vi "IV_config_DMM.vi"(8 "error in (no error)":errorcluster, 11 "Input parameters":T1={"Measurement type"=enum."Debug", "Sensor type"=enum."HPK_8in_271ch", "Identifier"="test.txt", "Open after execution?"=FALSE, "Plot after execution?"=FALSE, "Display channel"=0, "Voltage Delay (s)"=0.5, "Switch Delay (s)"=0.01, "VISA resource name source"="", "VISA resource name DMM"="", "VISA resource name LCR"="", "Compliance  Level (A)"=10.0, "Voltage Limit (V)"=1000.0, "Data storage location"="", "Scan voltages"="", "Use source as DMM?"=FALSE, "LCR signal frequenzy (Hz)"=10.0, "DMM device"=enum."Keithley2001", "Sampling number"=1, "Use env. sensors on"=enum."Sensirion sht1x/7x", "Switchboard Handle"=0, "Use Switchboard"=FALSE, "LCR signal voltage (V)"=10000.0, "Repeat"=1, "Scan voltages IV"="", "Scan voltages CV"="", "Hex pad numbers?"=FALSE, "Set measurement type"=enum."Debug", "Custom pad scan"="", "IV voltage Delay (s)"=0.5, "CV voltage Delay (s)"=0.5, "Needle measurement?"=FALSE, "Comments"="test.txt", "LCR signal frequenzy (kHz)"=10.0, "Compliance  Level (uA)"=10.0, "Open Correction Array"=array2304x3[6912 elements], "Current set voltage"=0.0, "Last set voltage"=0.0, "Current channel"=0, "Last OpenCorrection index"=-1, "Total curr/vltg every x steps"=10, "Current channel iteration"=0, "No CV corrections"=FALSE, "Mapfile"="", "Corrfile"="", "IV voltage file"=path "", "CV voltage file"=path "", "IV Switch Delay (s)"=0.01, "CV Switch Delay (s)"=0.01, "Invert polarity"=FALSE, "Set debug dirs"=FALSE, "Is n on p"=FALSE, "Source interlock?"=TRUE, "Voltage file used?"=FALSE, "Pad mask"="", "Mask pad above (uA)"=1.0, "LCR device"=enum."LCR_E4980", "Source device"=enum."Source_2410"} {"CV Switch Delay (s)" format="%#_13g"; "IV Switch Delay (s)" format="%#_13g"; "Last set voltage" format="%#_13g"; "Current set voltage" format="%#_13g"; "CV voltage Delay (s)" format="%#_13g"; "IV voltage Delay (s)" format="%#_13g"; "Voltage Limit (V)" format="%#_13g"; "Voltage Delay (s)" format="%#_13g"; "Switch Delay (s)" format="%#_13g"}) -> (0 "error out":errorcluster)   [LabVIEW 2016]
doc: "Sets configuration for DMM."
uses:
  input_params.ctl
  <instrlib>/ke2001/KE2001.LLB/Keith 2001 Reset / Preset.vi
  <instrlib>/Keithley 2450/Keithley 2450.lvlib
  <instrlib>/Keithley 6517/Keithley 6517.lvlib
  <instrlib>/Keithley 648X Series/Keithley 648X Series.lvlib
panel:
  out "VISA resource name out":refnum<visa-resource-name>
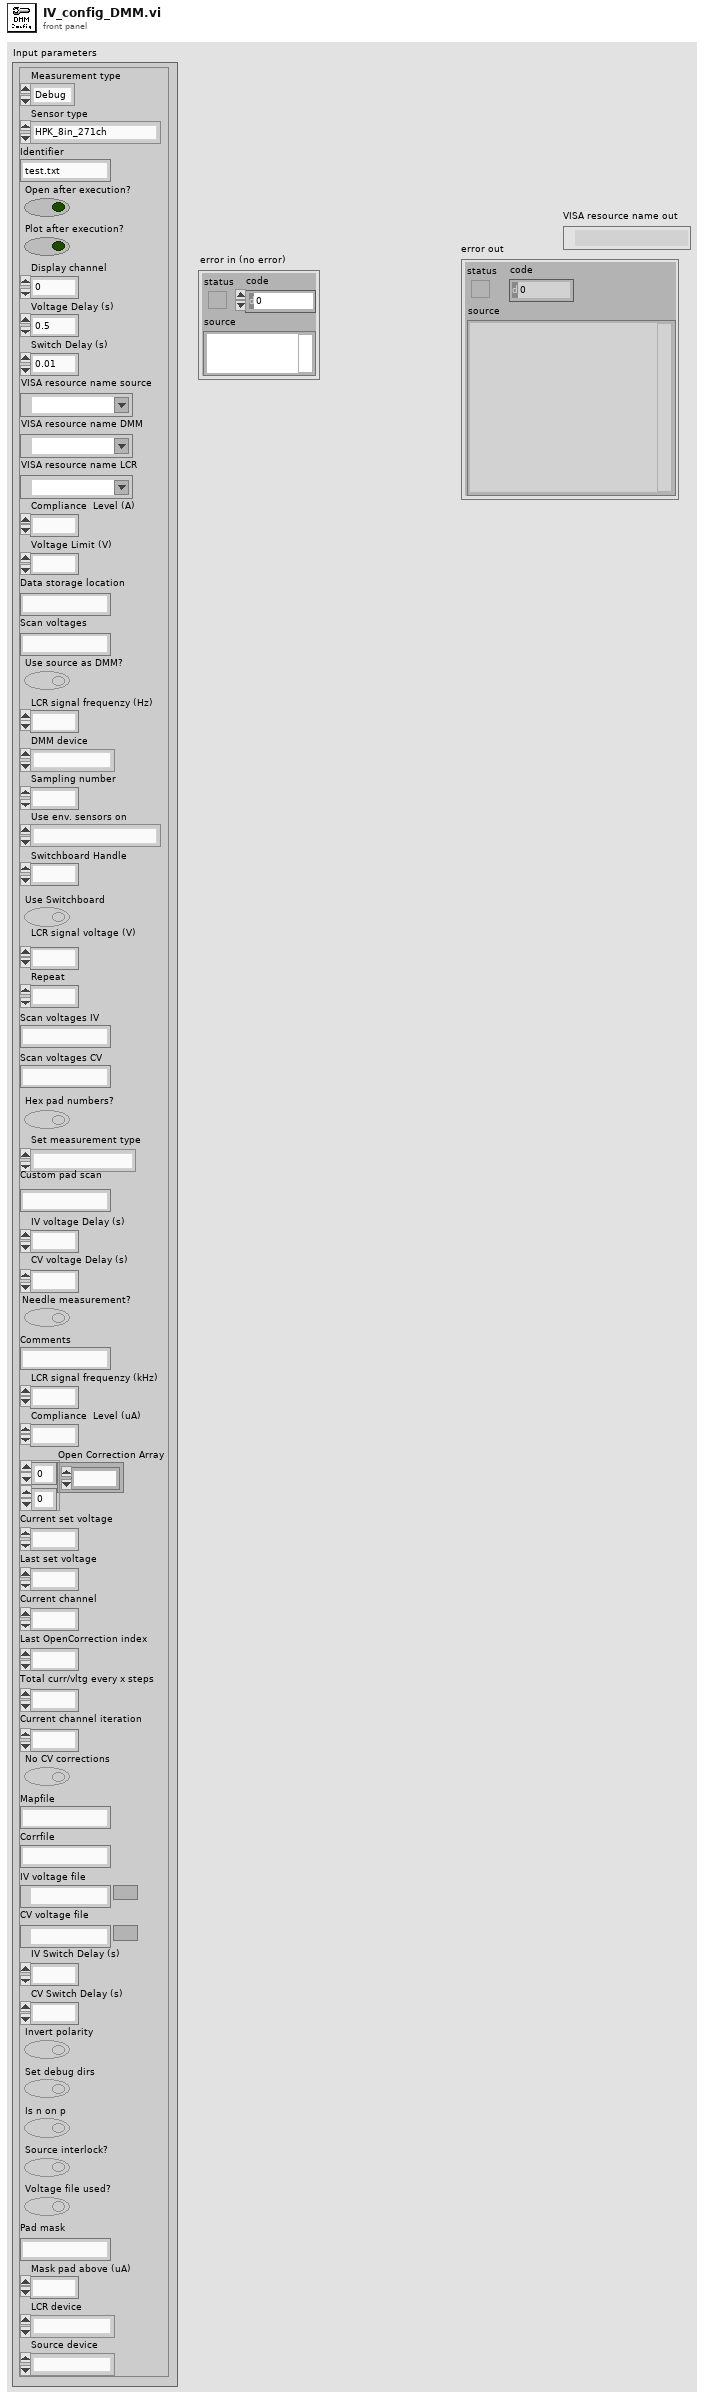
[diagram p1: front panel]
types:
  T1 = typedef "input_params.ctl" = cluster{"Measurement type":enum16{"IV", "CV", "Debug", "Test_contact"}, "Sensor type":enum16{"HPK_6in_135ch", "HPK_8in_271ch", "IFX_8in_256ch", "Diode", "HPK_6in_239ch", "Full_Matrix", "HPK_8in_271ch_full", "HPK_8in_198ch", "LumiCal"}, "Identifier":string, "Open after execution?":bool, "Plot after execution?":bool, "Display channel":i32, "Voltage Delay (s)":dbl, "Switch Delay (s)":dbl, "VISA resource name source":refnum<visa-resource-name>, "VISA resource name DMM":refnum<visa-resource-name>, "VISA resource name LCR":refnum<visa-resource-name>, "Compliance  Level (A)":dbl, "Voltage Limit (V)":dbl, "Data storage location":string, "Scan voltages":string, "Use source as DMM?":bool, "LCR signal frequenzy (Hz)":dbl, "DMM device":enum16{"Keithley2001", "Keithley2450", "Keithley2410", "Keithley6485", "Keithley6487", "Keithley6517"}, "Sampling number":i32, "Use env. sensors on":enum16{"Sensirion sht1x/7x", "Switch Matrix", "Probecard"}, "Switchboard Handle":u32, "Use Switchboard":bool, "LCR signal voltage (V)":dbl, "Repeat":i32, "Scan voltages IV":string, "Scan voltages CV":string, "Hex pad numbers?":bool, "Set measurement type":enum16{"IV", "CV", "Debug", "Test_contact", "IV+CV"}, "Custom pad scan":string, "IV voltage Delay (s)":dbl, "CV voltage Delay (s)":dbl, "Needle measurement?":bool, "Comments":string, "LCR signal frequenzy (kHz)":dbl, "Compliance  Level (uA)":dbl, "Open Correction Array":dbl[][], "Current set voltage":dbl, "Last set voltage":dbl, "Current channel":i32, "Last OpenCorrection index":i32, "Total curr/vltg every x steps":i32, "Current channel iteration":i32, "No CV corrections":bool, "Mapfile":string, "Corrfile":string, "IV voltage file":path, "CV voltage file":path, "IV Switch Delay (s)":dbl, "CV Switch Delay (s)":dbl, "Invert polarity":bool, "Set debug dirs":bool, "Is n on p":bool, "Source interlock?":bool, "Voltage file used?":bool, "Pad mask":string, "Mask pad above (uA)":dbl, "LCR device":enum16{"LCR_E4980", "AGILENT_4263X"}, "Source device":enum16{"Source_2410", "Source_6487"}}
  T2 = enum16{"Keithley2001", "Keithley2450", "Keithley2410", "Keithley6485", "Keithley6487", "Keithley6517"}
  T3 = enum16{"Auto On", "2e-9", "2e-8", "2e-7", "2e-6", "2e-5", "2e-4", "2e-3", "2e-2"}
  T4 = cluster{"error":bool, "code":i32, "source":string}
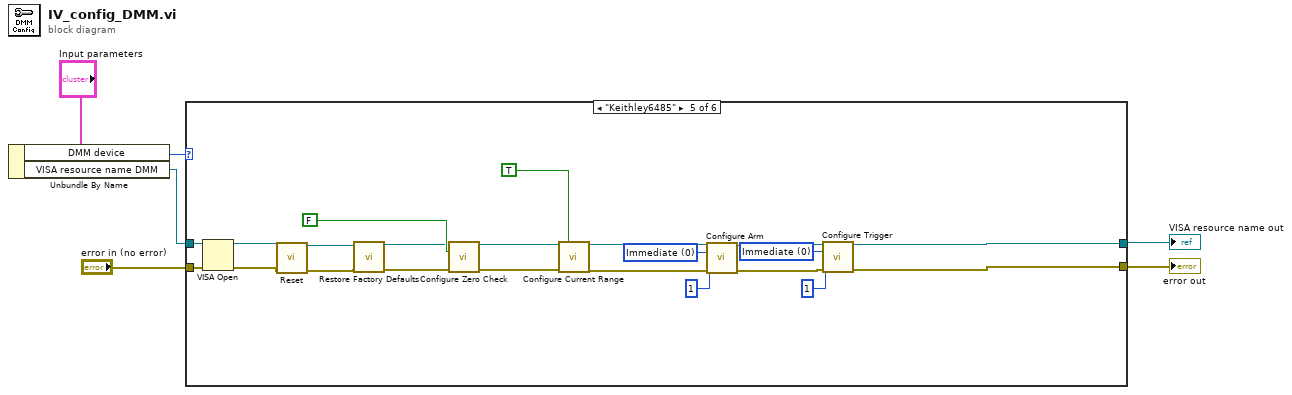
[diagram p0: block diagram]
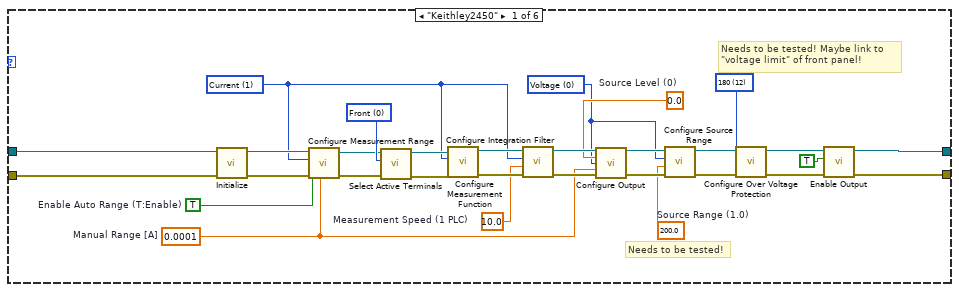
[diagram p2: hidden frame]
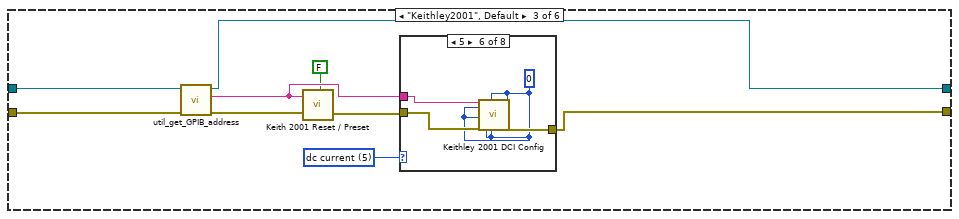
[diagram p4: hidden frame]
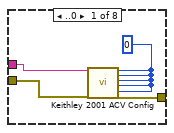
[diagram p5: hidden frame]
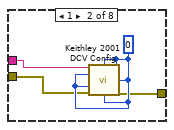
[diagram p6: hidden frame]
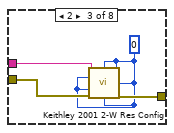
[diagram p7: hidden frame]
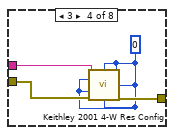
[diagram p8: hidden frame]
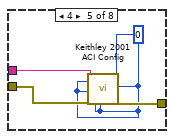
[diagram p9: hidden frame]
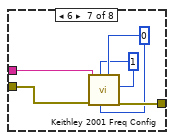
[diagram p10: hidden frame]
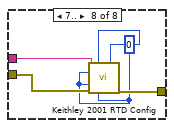
[diagram p11: hidden frame]
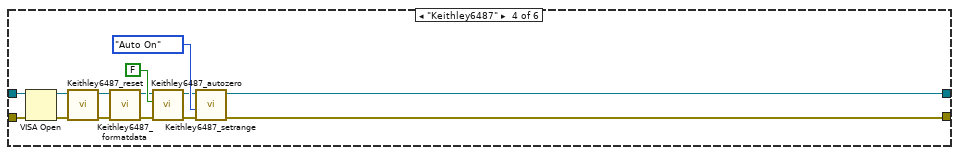
[diagram p12: hidden frame]
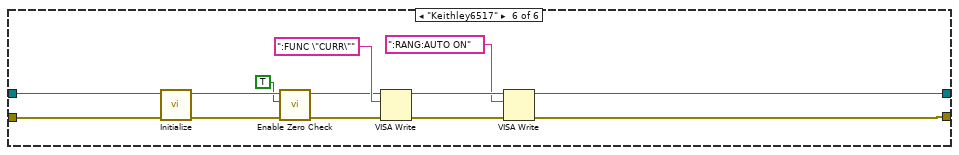
[diagram p13: hidden frame]
diagram:
  n1 = Unbundle By Name("Input parameters") -> ("DMM device"=w4:T2, "VISA resource name DMM"=w3:refnum<visa-resource-name>)
  n2 = case shown="\"Keithley6485\"" w4 {
    tunnel: w3 -> [w36 w38 w45 w83 w115 w123]
    tunnel: "error in (no error)" -> [w35 w37 w44 w84 w116 w122]
    tunnel: [w7 w37 w46 w85 w101 w118] -> w5
    tunnel: [w8 w38 w43 w86 w102 w119] -> w1
    frame "Keithley2450" {
      w12 = u16 12 items=["None", "2", "5", "10", "20", "40", "60", "80", "100", "120", "140", "160", "180"] ("Voltage Limit (0)")
      w15 = 200.0  # Source Range (1.0)
      w20 = 0.0  # Source Level (0)
      w16 = u16 0 items=["Voltage", "Current"] ("Source Mode  (0: Voltage)")
      w23 = 10.0  # Measurement Speed (1 PLC)
      w24 = u16 1 items=["Volts", "Current", "Resistance"] ("Function (0: Volts)")
      w19 = 0.0001  # Manual Range [A]
      w27 = TRUE  # Enable Auto Range (T:Enable)
      w32 = u16 0 items=["Front", "Rear"] ("Active Terminals (0: Front)")
      # "Needs to be tested! Maybe link to \n\"voltage limit\" of front panel!"
      # "Needs to be tested!"
      n3 = call <instrlib>:"Initialize.vi"("error in (no error)"=w35, "VISA resource name"=w36) -> ("error out"=w33:errorcluster, "VISA resource name out"=w34:refnum<visa-resource-name>)  [unwired: 8 in]
      n4 = call <instrlib>:"Configure Measurement Range.vi"("Manual Range (1.0)"=w19, "error in (no error)"=w33, "Enable Auto Range (T:Enable)"=w27, "Function (0: Volts)"=w24, "VISA resource name"=w34) -> ("error out"=w31:errorcluster, "VISA resource name out"=w28:refnum<visa-resource-name>)  [unwired: 5 in]
      n5 = call <instrlib>:"Select Active Terminals.vi"("error in (no error)"=w31, "Active Terminals (0: Front)"=w32, "VISA resource name"=w28) -> ("error out"=w30:errorcluster, "VISA resource name out"=w29:refnum<visa-resource-name>)  [unwired: 7 in]
      n6 = call <instrlib>:"Configure Measurement Function.vi"("error in (no error)"=w30, "Function (0: Volts)"=w24, "VISA resource name"=w29) -> ("error out"=w25:errorcluster, "VISA resource name out"=w26:refnum<visa-resource-name>)  [unwired: 7 in]
      n7 = call <instrlib>:"Configure Integration Filter.vi"("error in (no error)"=w25, "Measurement Speed (1 PLC)"=w23, "Function (0: Volts)"=w24, "VISA resource name"=w26) -> ("error out"=w21:errorcluster, "VISA resource name out"=w22:refnum<visa-resource-name>)  [unwired: 6 in]
      n8 = call <instrlib>:"Configure Output.vi"("VISA resource name"=w22, "Source Level (0)"=w20, "Source Mode  (0: Voltage)"=w16, "Source Limit Level (0.1)"=w19, "error in (no error)"=w21) -> ("VISA resource name out"=w17:refnum<visa-resource-name>, "error out"=w18:errorcluster)  [unwired: 9 in]
      n9 = call <instrlib>:"Configure Source Range.vi"("error in (no error)"=w18, "Source Range (1.0)"=w15, "Function (0: Volts)"=w16, "VISA resource name"=w17) -> ("error out"=w14:errorcluster, "VISA resource name out"=w13:refnum<visa-resource-name>)  [unwired: 6 in]
      n10 = call <instrlib>:"Configure Over Voltage Protection.vi"("error in (no error)"=w14, "Voltage Limit (0)"=w12, "VISA resource name"=w13) -> ("error out"=w10:errorcluster, "VISA resource name out"=w9:refnum<visa-resource-name>)  [unwired: 7 in]
      n11 = call <instrlib>:"Enable Output.vi"("error in (no error)"=w10, "Enable Output (T: Enable)"=TRUE, "VISA resource name"=w9) -> ("error out"=w7:errorcluster, "VISA resource name out"=w8:refnum<visa-resource-name>)  [unwired: 7 in]
    }
    frame "Keithley2410" {
    }
    frame "Keithley2001", Default {
      w47 = u16 5 items=["ac voltage", "dc voltage", "2-wire resistance", "4-wire resistance", "ac current", "dc current", "frequency", "temperature"] ("function (Vdc:1)")
      n12 = call "util_get_GPIB_address.vi"("error in (no error)"=w44, "VISA resource name"=w45) -> ("error out"=w42:errorcluster, "GPIB address"=w41:string, "VISA resource name out"=w43:refnum<visa-resource-name>)  [unwired: 7 in]
      n13 = call "Keith 2001 Reset / Preset.vi"("reset/preset"=FALSE, "error in"=w42, "GPIB address"=w41) -> ("error out"=w40:T4)
      n14 = case shown="5" w47 {
        tunnel: w40 -> [w50 w54 w58 w62 w66 w70 w75 w79]
        tunnel: w41 -> [w48 w53 w57 w61 w65 w68 w74 w78]
        tunnel: [w49 w52 w59 w63 w67 w71 w76 w80] -> w46
        frame ..0 {
          w51 = u16 0
          n15 = call <instrlib>:"Keithley 2001 ACV Config.vi"("GPIB address"=w48, "integration time (0:auto)"=w51, "integ. value"=w51, "range (auto:0)"=w51, "error in"=w50, "resolution (4.5 digits:3)"=w51, "reference (off:0)"=w51, "digital filter (off:0)"=w51, "advanced filter (off:0)"=w51, "detector (rms:0)"=w51) -> ("error out"=w49:T4)  [unwired: 9 in]
        }
        frame 1 {
          w55 = u16 0
          n16 = call <instrlib>:"Keithley 2001 DCV Config.vi"("GPIB address"=w53, "range (auto:0)"=w55, "digital filter (off:0)"=w55, "integration time (0:auto)"=w55, "advanced filter (off:0)"=w55, "resolution (4.5 digits:3)"=w55, "error in"=w54, "reference value (volts)"=w55) -> ("error out"=w52:T4)  [unwired: 7 in]
        }
        frame 2 {
          w56 = u16 0
          n17 = call <instrlib>:"Keithley 2001 2-W Res Config.vi"("GPIB address"=w57, "range (auto:0)"=w56, "digital filter (off:0)"=w56, "integration time (0:auto)"=w56, "advanced filter (off:0)"=w56, "resolution (4.5 digits:3)"=w56, "error in"=w58, "reference value (ohms)"=w56) -> ("error out"=w59:T4)  [unwired: 7 in]
        }
        frame 3 {
          w60 = u16 0
          n18 = call <instrlib>:"Keithley 2001 4-W Res Config.vi"("GPIB address"=w61, "range (auto:0)"=w60, "digital filter (off:0)"=w60, "integration time (0:auto)"=w60, "advanced filter (off:0)"=w60, "resolution (4.5 digits:3)"=w60, "error in"=w62, "reference value (ohms)"=w60) -> ("error out"=w63:T4)  [unwired: 7 in]
        }
        frame 4 {
          w64 = u16 0
          n19 = call <instrlib>:"Keithley 2001 ACI Config.vi"("GPIB address"=w65, "integration time (0:auto)"=w64, "range (auto:0)"=w64, "error in"=w66, "resolution (4.5 digits:3)"=w64, "digital filter (off:0)"=w64, "advanced filter (off:0)"=w64, "detector (rms:0)"=w64) -> ("error out"=w67:T4)  [unwired: 11 in]
        }
        frame 5 {
          w69 = u16 0
          n20 = call <instrlib>:"Keithley 2001 DCI Config.vi"("GPIB address"=w68, "integration time (0:auto)"=w69, "range (auto:0)"=w69, "error in"=w70, "resolution (4.5 digits:3)"=w69, "reference (off:0)"=w69, "digital filter (off:0)"=w69, "advanced filter (off:0)"=w69) -> ("error out"=w71:T4)  [unwired: 11 in]
        }
        frame 6 {
          w72 = u16 1
          w73 = u16 0
          n21 = call <instrlib>:"Keithley 2001 Freq Config.vi"("threshold voltage range (10V:1)"=w72, "threshold current range (1mA:0)"=w73, "reference (off:0)"=w73, "resolution (5 digits:1)"=w72, "error in"=w75, "GPIB address"=w74) -> ("error out"=w76:T4)  [unwired: 5 in]
        }
        frame 7.. {
          w77 = u16 0
          n22 = call <instrlib>:"Keithley 2001 RTD Config.vi"("GPIB address"=w78, "reference (off:0)"=w77, "transducer (2-W RTD-PT385:0)"=w77, "integration time (0:auto)"=w77, "resolution (5.5 digits:4)"=w77, "error in"=w79, "digital filter (off:0)"=w77) -> ("error out"=w80:T4)  [unwired: 8 in]
        }
      }
    }
    frame "Keithley6487" {
      n23 = VISA Open(error in (no error)=w84, VISA resource name=w83) -> (VISA resource name=w82:refnum<visa-resource-name>, error out=w81:errorcluster)  [unwired: 3 in]
      n24 = call <instrlib>:"Keithley6487_reset.vi"("error in (no error)"=w81, "VISA resource name"=w82) -> ("error out"=w92:errorcluster, "VISA resource name out"=w89:refnum<visa-resource-name>)  [unwired: 8 in]
      n25 = call <instrlib>:"Keithley6487_formatdata.vi"("error in (no error)"=w92, "VISA resource name"=w89) -> ("error out"=w91:errorcluster, "VISA resource name out"=w88:refnum<visa-resource-name>)  [unwired: 8 in]
      n26 = call <instrlib>:"Keithley6487_autozero.vi"("error in (no error)"=w91, "Autozero"=FALSE, "VISA resource name"=w88) -> ("error out"=w90:errorcluster, "VISA resource name out"=w87:refnum<visa-resource-name>)  [unwired: 7 in]
      n27 = call <instrlib>:"Keithley6487_setrange.vi"("error in (no error)"=w90, "Enum"=T3."Auto On", "VISA resource name"=w87) -> ("error out"=w85:errorcluster, "VISA resource name out"=w86:refnum<visa-resource-name>)  [unwired: 7 in]
    }
    frame "Keithley6485" {
      w96 = u16 0 items=["Immediate", "Tlink"] ("Trigger Source (0: Immediate)")
      w98 = u16 0 items=["Immediate", "Timer", "Bus", "Tlink", "Manual", "Negative SOT", "Positive SOT", "Bidirectional SOT"] ("Arm Source (0: Immediate)")
      n28 = VISA Open(error in (no error)=w116, VISA resource name=w115) -> (VISA resource name=w113:refnum<visa-resource-name>, error out=w114:errorcluster)  [unwired: 3 in]
      n29 = call <instrlib>:"Reset.vi"("VISA resource name"=w113, "error in (no error)"=w114) -> ("VISA resource name out"=w112:refnum<visa-resource-name>, "error out"=w111:errorcluster)  [unwired: 12 in]
      n30 = call <instrlib>:"Restore Factory Defaults.vi"("VISA resource name"=w112, "error in (no error)"=w111) -> ("VISA resource name out"=w109:refnum<visa-resource-name>, "error out"=w108:errorcluster)  [unwired: 12 in]
      n31 = call <instrlib>:"Configure Zero Check.vi"("VISA resource name"=w109, "Enable Zero Check (T: Enable)"=FALSE ("Autozero"), "error in (no error)"=w108) -> ("VISA resource name out"=w106:refnum<visa-resource-name>, "error out"=w105:errorcluster)  [unwired: 11 in]
      n32 = call <instrlib>:"Configure Current Range.vi"("VISA resource name"=w106, "Autorange (T: Enable)"=TRUE, "error in (no error)"=w105) -> ("VISA resource name out"=w104:refnum<visa-resource-name>, "error out"=w99:errorcluster)  [unwired: 11 in]
      n33 = call <instrlib>:"Configure Arm.vi"("VISA resource name"=w104, "Arm Source (0: Immediate)"=w98, "Arm Loop Count (1)"=1, "error in (no error)"=w99) -> ("VISA resource name out"=w103:refnum<visa-resource-name>, "error out"=w100:errorcluster)  [unwired: 10 in]
      n34 = call <instrlib>:"Configure Trigger.vi"("VISA resource name"=w103, "Trigger Source (0: Immediate)"=w96, "Trigger Loop Count (1)"=1, "error in (no error)"=w100) -> ("VISA resource name out"=w102:refnum<visa-resource-name>, "error out"=w101:errorcluster)  [unwired: 10 in]
    }
    frame "Keithley6517" {
      n35 = call <instrlib>:"Initialize.vi"("error in (no error)"=w122, "VISA resource name"=w123) -> ("error out"=w128:errorcluster, "VISA resource name out"=w126:refnum<visa-resource-name>)  [unwired: 8 in]
      n36 = call <instrlib>:"Enable Zero Check.vi"("error in (no error)"=w128, "Enable Zero Check (T: Enable)"=TRUE, "VISA resource name"=w126) -> ("error out"=w127:errorcluster, "VISA resource name out"=w125:refnum<visa-resource-name>)  [unwired: 7 in]
      n37 = VISA Write(VISA resource name=w125, write buffer=":FUNC \"CURR\"", error in (no error)=w127) -> (VISA resource name out=w121:refnum<visa-resource-name>, error out=w120:errorcluster)  [unwired: 1 out]
      n38 = VISA Write(VISA resource name=w121, write buffer=":RANG:AUTO ON", error in (no error)=w120) -> (VISA resource name out=w119:refnum<visa-resource-name>, error out=w118:errorcluster)  [unwired: 1 out]
    }
  }
  "VISA resource name out" <- w1
  "error out" <- w5
